vi "Generic DAQmx DIO Shutter Engine.vi"(0 "Unique Notifier Name":string="Not a Name", 11 "DIO Lines":string[](array[string])) -> ()   [LabVIEW 2016]
uses:
  Shutter Controls/Shutter Notifier Element.ctl
  Shutter Controls/Shutter Actions.ctl
  <vilib>/DAQmx/write.llb/DAQmx Write (Digital Bool 1Line 1Point).vi
  <vilib>/DAQmx/read.llb/DAQmx Read (Digital Bool 1Line 1Point).vi
  <vilib>/DAQmx/create/channels.llb/DAQmx Create Channel (DO-Digital Output).vi
  <vilib>/DAQmx/miscellaneous.llb/DAQmx Fill In Error Info.vi
  <vilib>/DAQmx/create/channels.llb/DAQmx Create Channel (DI-Digital Input).vi
panel:
  in  "Quit":bool
  in  "Shutter":bool
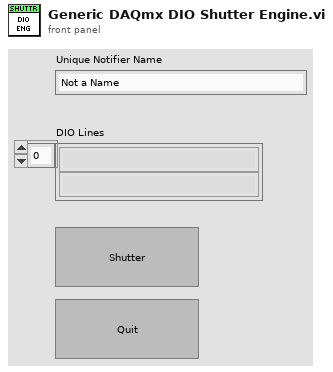
[diagram p1: front panel]
types:
  T1 = typedef "Shutter Notifier Element.ctl" = cluster{"Action":T2, "Status":T2, "Received?":bool}
  T2 = typedef "Shutter Actions.ctl" = enum16{"Open", "Close", "Toggle", "Status", "Quit"}
  T3 = enum32{"Invalid", "Standard", "Closed", "Hidden", "Minimized", "Maximized"}
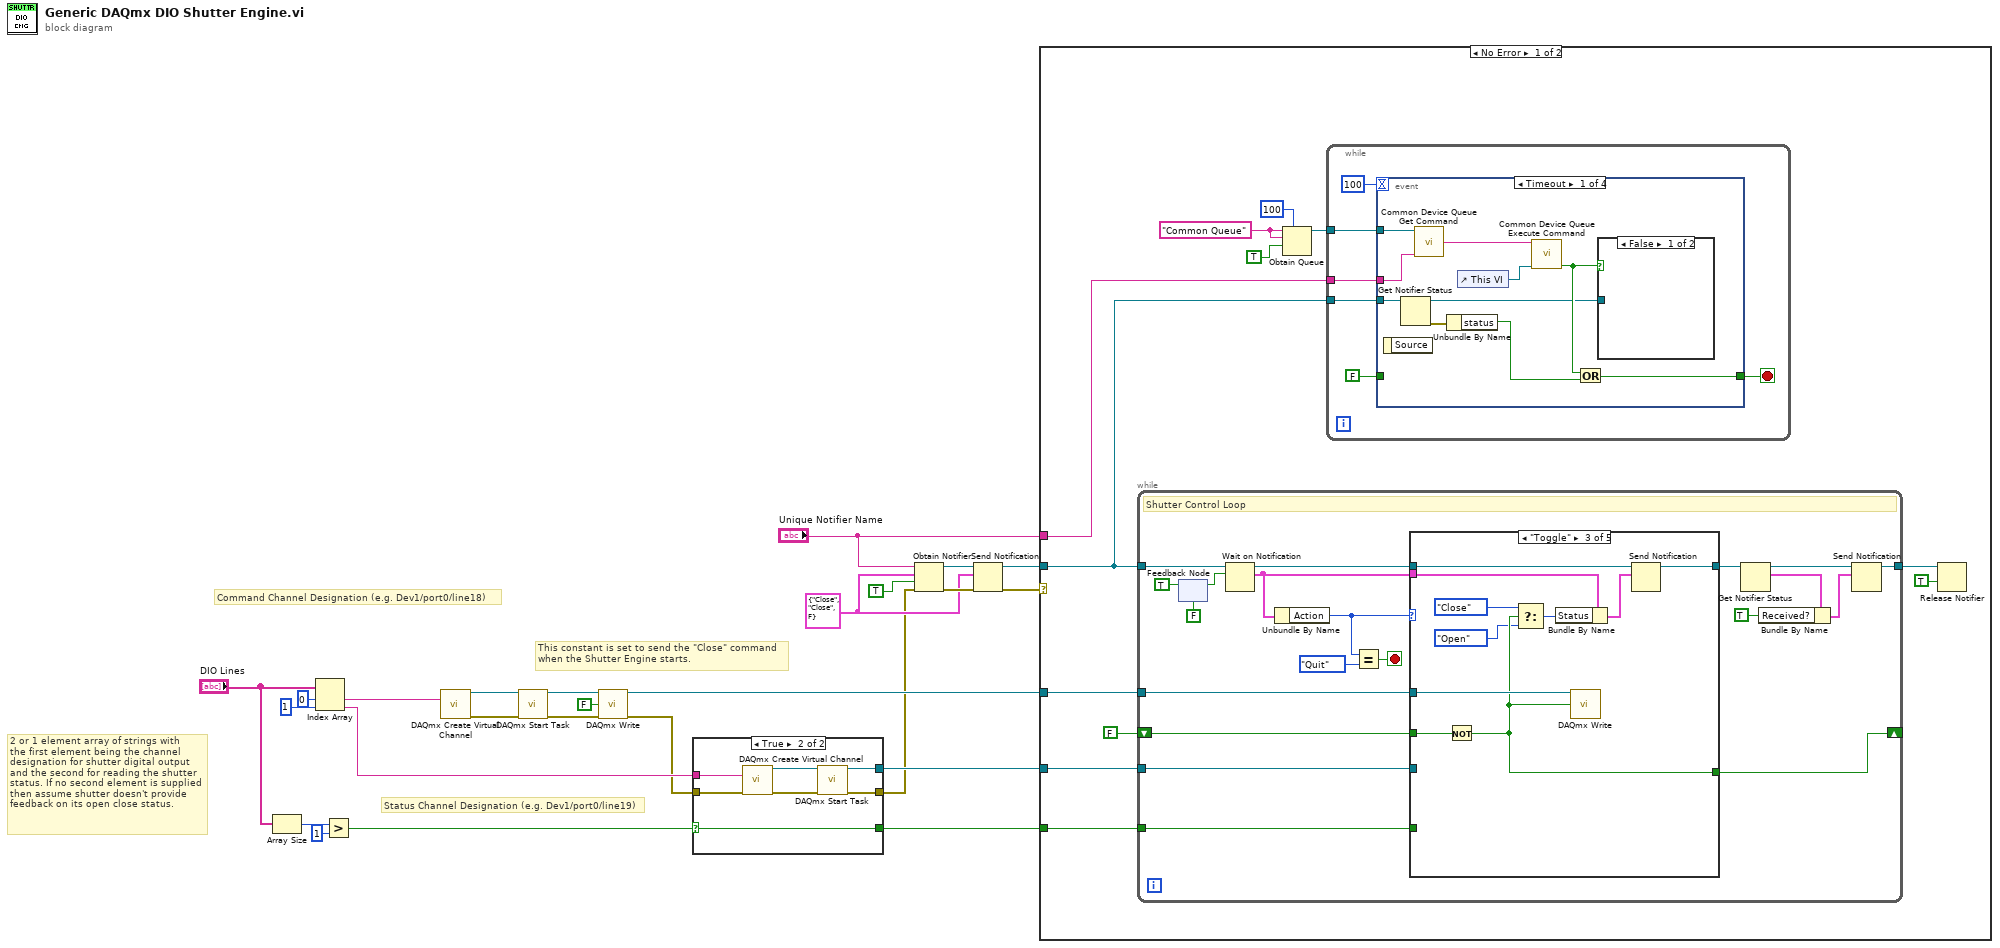
[diagram p0: block diagram]
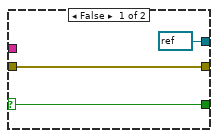
[diagram p2: hidden frame]
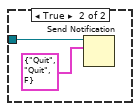
[diagram p3: hidden frame]
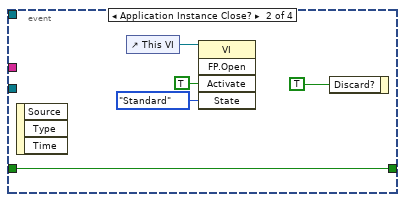
[diagram p4: hidden frame]
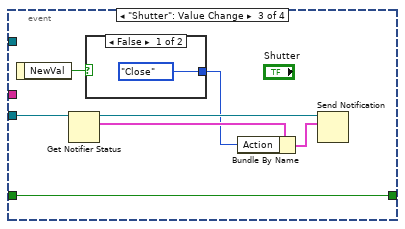
[diagram p5: hidden frame]
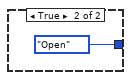
[diagram p6: hidden frame]
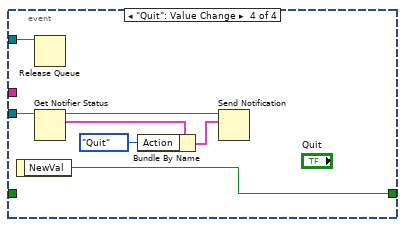
[diagram p7: hidden frame]
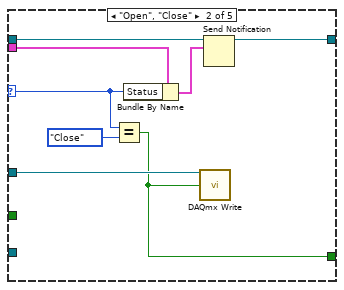
[diagram p9: hidden frame]
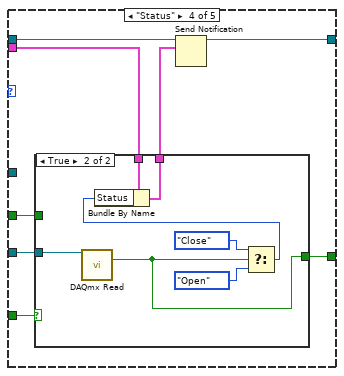
[diagram p10: hidden frame]
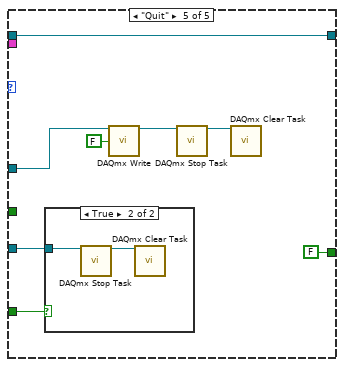
[diagram p12: hidden frame]
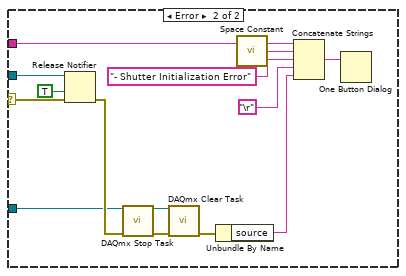
[diagram p14: hidden frame]
diagram:
  w15 = T1 {"Action"=enum."Close", "Status"=enum."Close", "Received?"=FALSE} ("Shutter Notifier Element")
  # "This constant is set to send the \"Close\" command\nwhen the Shutter Engine starts."
  # "2 or 1 element array of strings with\nthe first element being the channel\ndesignation for shutter digital output\nand the second for reading the shutter\nstatus. If no second element is supplied\nthen assume shutter doesn't provide\nfeedback on its open close status."
  # "Status Channel Designation (e.g. Dev1/port0/line19)"
  # "Command Channel Designation (e.g. Dev1/port0/line18)"
  n1 = Array Size(array="DIO Lines") -> (size(s)=w7:i32)
  n2 = Index Array(array="DIO Lines", index #1=0 ("index"), index #2=1 ("index")) -> (element #1=w1:string, element #2=w9:string)
  n3 = Greater?(x=w7, y=1) -> (0:w3:bool)
  n4 = call-poly <vilib>:"DAQmx Create Virtual Channel.vi"("lines"=w1) -> ("task out"=w24:refnum<k21>, "error out"=w25:errorcluster)  [unwired: 4 in, 9 out]
  n5 = call <vilib>:"DAQmx Start Task.vi"("task/channels in"=w24, "error in"=w25) -> ("task out"=w19:refnum<k21>, "error out"=w20:errorcluster)  [unwired: 12 out]
  n6 = call-poly <vilib>:"DAQmx Write.vi"("task/channels in"=w19, "data"=FALSE, "error in"=w20) -> ("task out"=w17:refnum<k21>, "error out"=w5:errorcluster)  [unwired: 1 in, 10 out]
  n7 = case shown="True" w3 {
    selector: w3 -> [w26 w29]
    tunnel: [refnum<k21> refnum ("task out") w33] -> w14
    tunnel: w9 -> [_ w32]
    tunnel: w5 -> [w27 w31]
    tunnel: [w27 w30] -> w4
    tunnel: [w26 w29] -> w2
    frame False {
    }
    frame True {
      n8 = call-poly <vilib>:"DAQmx Create Virtual Channel.vi"("lines"=w32, "error in"=w31) -> ("task out"=w35:refnum<k21>, "error out"=w34:errorcluster)  [unwired: 3 in, 9 out]
      n9 = call <vilib>:"DAQmx Start Task.vi"("task/channels in"=w35, "error in"=w34) -> ("task out"=w33:refnum<k21>, "error out"=w30:errorcluster)  [unwired: 12 out]
    }
  }
  n10 = Obtain Notifier(name (unnamed)="Unique Notifier Name", notification data type=w15, create if not found? (T)=TRUE, error in (no error)=w4) -> (notifier out=w22:refnum<notifier>, error out=w21:errorcluster)  [unwired: 1 out]
  n11 = Send Notification(notification=w15, notifier=w22, error in (no error)=w21) -> (notifier out=w16:refnum<notifier>, error out=w13:errorcluster)
  n12 = case shown="No Error" w13 {
    selector: w13 -> [_ w160]
    tunnel: w17 -> [w47 w162]
    tunnel: w16 -> [w42 w163]
    tunnel: w14 -> [w44 _]
    tunnel: "Unique Notifier Name" -> [w41 w159]
    tunnel: w2 -> [w43 _]
    frame No Error {
      w39 = "Common Queue" ("Unique Notifier Name")
      n13 = while {
        tunnel: w42 -> [w96]
        tunnel: w47 -> [w104]
        tunnel: [w98] -> w45
        tunnel: w44 -> [w97]
        tunnel: w43 -> [w89]
        shift-right: [w87] -> _
        shift-left: FALSE -> [w88]
        stop <- w105 stop-if-true
        # "Shutter Control Loop"
        n14 = feedback #1(FALSE) -> (w92:bool)
        n15 = feedback-in #1(TRUE) -> ()
        n16 = Wait on Notification(notifier=w96, ignore previous (F)=w92) -> (notifier out=w95:refnum<notifier>, notification=w91:T1)  [unwired: 2 in, 2 out]
        n17 = Unbundle By Name(w91) -> ("Action"=w90:T2)
        n18 = Equal?(x=w90, y=Shutter_Actions."Quit") -> (x = y?=w105:bool)
        n19 = case shown="\"Toggle\"" w90 {
          selector: w90 -> [_ w110 _ _ _]
          tunnel: w95 -> [w108 w113 w123 w130 w151]
          tunnel: w104 -> [_ w114 w126 _ w149]
          tunnel: [w108 w115 w122 w132 w151] -> w101
          tunnel: w97 -> [_ _ _ w134 w146]
          tunnel: w91 -> [_ w112 w121 w131 _]
          tunnel: w89 -> [_ _ _ w129 w145]
          tunnel: w88 -> [w107 _ w125 w128 _]
          tunnel: [w107 w109 w120 w127 FALSE ("data")] -> w87
          frame Default {
          }
          frame "Open", "Close" {
            n20 = Equal?(x=w110, y=Shutter_Actions."Close") -> (x = y?=w109:bool)
            n21 = Bundle By Name(cluster=w112, "Status"=w110) -> (w116:T1)
            n22 = call-poly <vilib>:"DAQmx Write.vi"("task/channels in"=w114, "data"=w109) -> ()  [unwired: 2 in, 12 out]
            n23 = Send Notification(notification=w116, notifier=w113) -> (notifier out=w115:refnum<notifier>)  [unwired: 1 in, 1 out]
          }
          frame "Toggle" {
            n24 = Not(x=w125) -> (.not. x?=w120:bool)
            n25 = Select(t=Shutter_Actions."Close" ("Status"), s=w120, f=Shutter_Actions."Open" ("Status")) -> (s? t:f=w117:T2)
            n26 = Bundle By Name(cluster=w121, "Status"=w117) -> (w124:T1)
            n27 = call-poly <vilib>:"DAQmx Write.vi"("task/channels in"=w126, "data"=w120) -> ()  [unwired: 2 in, 12 out]
            n28 = Send Notification(notification=w124, notifier=w123) -> (notifier out=w122:refnum<notifier>)  [unwired: 1 in, 1 out]
          }
          frame "Status" {
            n29 = case shown="True" w129 {
              tunnel: w134 -> [_ w143]
              tunnel: [w136 w140] -> w133
              tunnel: w131 -> [w136 w138]
              tunnel: w128 -> [w135 _]
              tunnel: [w135 w137] -> w127
              frame False {
              }
              frame True {
                n30 = call-poly <vilib>:"DAQmx Read.vi"("task/channels in"=w143) -> ("data"=w137:bool)  [unwired: 12 in, 2 out]
                n31 = Select(t=Shutter_Actions."Close" ("Shutter Status"), s=w137, f=Shutter_Actions."Open" ("Shutter Status")) -> (s? t:f=w139:T2)
                n32 = Bundle By Name(cluster=w138, "Status"=w139) -> (w140:T1)
              }
            }
            n33 = Send Notification(notification=w133, notifier=w130) -> (notifier out=w132:refnum<notifier>)  [unwired: 1 in, 1 out]
          }
          frame "Quit" {
            n34 = case shown="True" w145 {
              tunnel: w146 -> [_ w153]
              frame False {
              }
              frame True {
                n35 = call <vilib>:"DAQmx Stop Task.vi"("task/channels in"=w153) -> ("task out"=w152:refnum<k21>)  [unwired: 13 in, 1 out]
                n36 = call <vilib>:"DAQmx Clear Task.vi"("task in"=w152) -> ()  [unwired: 1 in, 14 out]
              }
            }
            n37 = call-poly <vilib>:"DAQmx Write.vi"("task/channels in"=w149, "data"=FALSE) -> ("task out"=w147:refnum<k21>)  [unwired: 2 in, 11 out]
            n38 = call <vilib>:"DAQmx Stop Task.vi"("task/channels in"=w147) -> ("task out"=w148:refnum<k21>)  [unwired: 13 in, 1 out]
            n39 = call <vilib>:"DAQmx Clear Task.vi"("task in"=w148) -> ()  [unwired: 1 in, 14 out]
          }
        }
        n40 = Get Notifier Status(notifier=w101) -> (notifier out=w99:refnum<notifier>, current notification=w102:T1)  [unwired: 1 in, 3 out]
        n41 = Bundle By Name(cluster=w102, "Received?"=TRUE) -> (w103:T1)
        n42 = Send Notification(notification=w103, notifier=w99) -> (notifier out=w98:refnum<notifier>)  [unwired: 1 in, 1 out]
      }
      n43 = Obtain Queue(max queue size (-1, unlimited)=100, name (unnamed)=w39, element data type=w39, create if not found? (T)=TRUE) -> (queue out=w36:refnum<queue>)  [unwired: 1 in, 2 out]
      n44 = while {
        tunnel: w36 -> [w53]
        tunnel: w42 -> [w50]
        tunnel: w41 -> [w48]
        stop <- w49 stop-if-true
        n45 = event shown="[0] Timeout" {
          selector: _ -> [_ _ _ _]
          dyn-events: _ -> [_ _ _ _]
          timeout: 100 -> [_ _ _ _]
          tunnel: w53 -> [w61 _ _ w80]
          tunnel: FALSE -> [_ w70 w73 _]
          tunnel: w50 -> [w63 _ w77 w81]
          tunnel: [w56 w70 w73 w86] -> w49
          tunnel: w48 -> [w60 _ _ _]
          event Timeout {
            n46 = event-data() -> ()  [unwired: 1 in, 1 out]
            n47 = Get Notifier Status(notifier=w63) -> (notifier out=w54:refnum<notifier>, error out=w62:errorcluster)  [unwired: 1 in, 3 out]
            n48 = call "Common Device Queue Get Command.vi"("Common Queue"=w61, "Notifier Name"=w60) -> ("Command"=w59:string)  [unwired: 12 in, 1 out]
            n49 = Unbundle By Name(w62) -> ("status"=w57:bool)
            n50 = control-ref of="This VI"() -> (w58:refnum<vi>)
            n51 = call "Common Device Queue Execute Command.vi"("Common Command"=w59, "VI Refnum"=w58) -> ("Quit?"=w55:bool)  [unwired: 12 in, 1 out]
            n52 = Or(x=w55, y=w57) -> (x .or. y?=w56:bool)
            n53 = case shown="False" w55 {
              tunnel: w54 -> [_ w65]
              frame False {
              }
              frame True {
                n54 = Send Notification(notification=T1 {"Action"=enum."Quit", "Status"=enum."Quit", "Received?"=FALSE} ("Shutter Notifier Element"), notifier=w65) -> ()  [unwired: 1 in, 2 out]
              }
            }
          }
          event Application Instance Close? {
            n55 = event-data() -> ()  [unwired: 1 in, 3 out]
            n56 = control-ref of="This VI"() -> (w67:refnum<vi>)
            n57 = invoke class="VI" method="FP.Open"(reference=w67, "Activate"=TRUE ("Activate?"), "State"=T3."Standard") -> ()  [unwired: 2 in, 5 out]
            n58 = event-data("Discard?"=TRUE) -> ()  [unwired: 1 in, 1 out]
          }
          event "Shutter": Value Change {
            n59 = event-data() -> ("NewVal"=w72:bool)  [unwired: 1 in]
            n60 = Get Notifier Status(notifier=w77) -> (notifier out=w76:refnum<notifier>, current notification=w75:T1)  [unwired: 1 in, 3 out]
            n61 = case shown="False" w72 {
              tunnel: [Shutter_Actions."Close" ("Action") Shutter_Actions."Open" ("Action")] -> w71
              frame False {
              }
              frame True {
              }
            }
            n62 = Bundle By Name(cluster=w75, "Action"=w71) -> (w74:T1)
            n63 = Send Notification(notification=w74, notifier=w76) -> ()  [unwired: 1 in, 2 out]
          }
          event "Quit": Value Change {
            n64 = event-data() -> ("NewVal"=w86:bool)  [unwired: 1 in]
            n65 = Release Queue(queue=w80) -> ()  [unwired: 2 in, 3 out]
            n66 = Get Notifier Status(notifier=w81) -> (notifier out=w85:refnum<notifier>, current notification=w84:T1)  [unwired: 1 in, 3 out]
            n67 = Bundle By Name(cluster=w84, "Action"=Shutter_Actions."Quit") -> (w83:T1)
            n68 = Send Notification(notification=w83, notifier=w85) -> ()  [unwired: 1 in, 2 out]
          }
        }
      }
      n69 = Release Notifier(notifier=w45, force destroy? (F)=TRUE) -> ()  [unwired: 1 in, 3 out]
    }
    frame Error {
      n70 = Release Notifier(notifier=w163, force destroy? (F)=TRUE, error in (no error)=w160) -> (error out=w164:errorcluster)  [unwired: 2 out]
      n71 = call <vilib>:"DAQmx Stop Task.vi"("task/channels in"=w162, "error in"=w164) -> ("task out"=w166:refnum<k21>, "error out"=w165:errorcluster)  [unwired: 12 in]
      n72 = call <vilib>:"DAQmx Clear Task.vi"("task in"=w166, "error in"=w165) -> ("error out"=w161:errorcluster)  [unwired: 13 out]
      n73 = Unbundle By Name(w161) -> ("source"=w154:string)
      n74 = call <vilib>:"Space Constant.vi"() -> ("String"=w157:string)
      n75 = Concatenate Strings(w159, w157, "- Shutter Initialization Error" ("string"), "\r", w154) -> (w158:string)
      n76 = One Button Dialog(message=w158) -> ()  [unwired: 1 in, 1 out]
    }
  }
